vi "Get Send Type.vi"(11 "Coupled Message Scripter in":refnum<class "Coupled Message Scripter.lvclass">) -> (2 "Send Type":enum16{"Concrete", "Abstract"}(ring))   [LabVIEW 2020, in "Message Maker.lvlib" / "Coupled Message Scripter.lvclass"]
uses:
  Coupled Message Scripter.lvclass
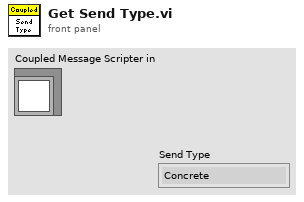
[diagram p1: front panel]
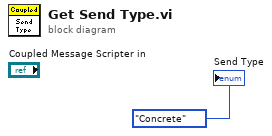
[diagram p0: block diagram]
diagram:
  "Send Type" <- enum16{"Concrete", "Abstract"}."Concrete" ("Send Type")
